vi "BRig_Host_dataRunState_idx_init.vi"() -> (2 "output_idx":i32[](array[numeric]))   [LabVIEW 2014]
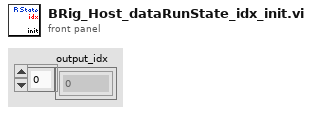
[diagram p1: front panel]
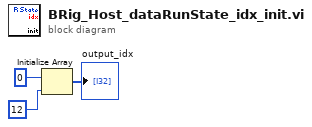
[diagram p0: block diagram]
diagram:
  n1 = Initialize Array(0 ("element"), 12 ("dimension size")) -> (→"output_idx":i32[])
